vi "I2C_Detect Example.vi"(5 "Bus":i32=1, 6 "error in":errorcluster) -> (0 "error out":errorcluster, 4 "I2C Devices":u8[](array[numeric]) format="%.0x")   [LabVIEW 2014]
doc: "Scans for I2C devices on the specified bus.\n\nThis VI uses the same technique as the i2cdetect tool, consult the documentation for the known issues."
uses:
  GPIO.lvlib
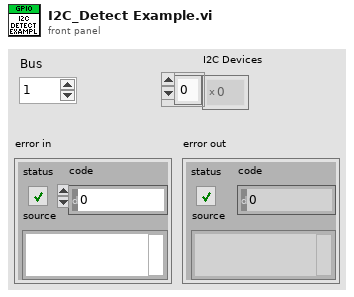
[diagram p1: front panel]
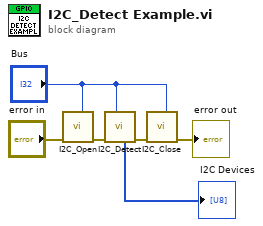
[diagram p0: block diagram]
diagram:
  n1 = call "I2C_Open.vi"("Bus"="Bus", "error in"="error in") -> ("error out"=w3:errorcluster)  [unwired: 9 in]
  n2 = call "I2C_Detect.vi"("Bus"="Bus", "error in"=w3) -> ("error out"=w5:errorcluster, "I2C Devices"=→"I2C Devices":u8[])  [unwired: 6 in]
  n3 = call "I2C_Close.vi"("Bus"="Bus", "error in"=w5) -> ("error out"=→"error out":errorcluster)  [unwired: 9 in]
